vi "Read Spec Page Path.vi"(8 "error in":errorcluster, 11 "DecideProjectFeatures In":refnum<class "editorscriptingobjectBasicExec.lvclass">) -> (0 "error out":errorcluster, 2 "Path to Spec Page VI":path, 3 "DecideProjectFeatures Out":refnum<class "editorscriptingobjectBasicExec.lvclass">)   [LabVIEW 2013, in "editorscriptingobjectBasicExec.lvclass"]
uses:
  editorscriptingobjectBasicExec.lvclass
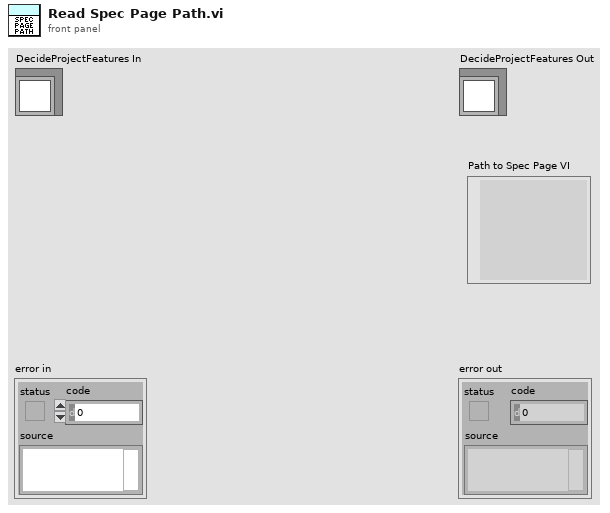
[diagram p1: front panel]
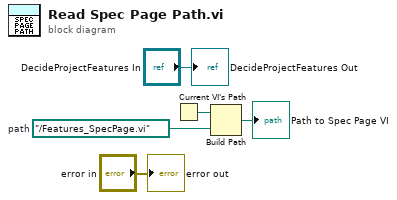
[diagram p0: block diagram]
diagram:
  w2 = path "../Features_SpecPage.vi"  # path
  n1 = Current VI's Path() -> (path=w3:path)
  n2 = Build Path(base path=w3, name or relative path=w2) -> (appended path=→"Path to Spec Page VI":path)
  "error out" <- "error in"
  "DecideProjectFeatures Out" <- "DecideProjectFeatures In"
